vi "FiltroHSV.vi"(8 "error in (no error)":errorcluster, 11 "Refnum in":T1) -> (3 "Array":u32[][](array[numeric]))   [LabVIEW 2021]
uses:
  <vilib>/vision/Image Controls.llb/IMAQ Image.ctl
  <vilib>/vision/NI_Vision_Development_Module.lvlib
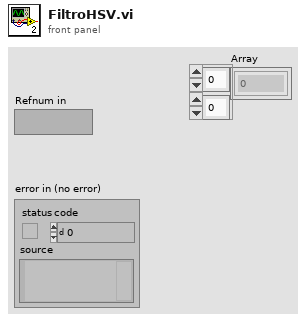
[diagram p1: front panel]
types:
  T1 = typedef "IMAQ Image.ctl" = refnum<image>
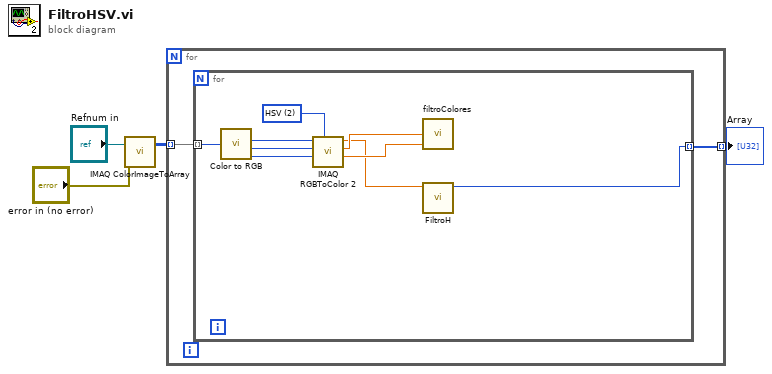
[diagram p0: block diagram]
diagram:
  n1 = call "IMAQ ColorImageToArray"("Image"="Refnum in", "error in (no error)"="error in (no error)") -> ("Image Pixels (U32)"=w1:u32[][])  [unwired: 2 in, 2 out]
  n2 = for {
    tunnel: w1 -> [w6] mode=indexing
    tunnel: [w5] -> w4 mode=indexing
    n3 = for {
      tunnel: w6 -> [w11] mode=indexing
      tunnel: [w7] -> w5 mode=indexing
      w12 = u16 2 items=["RGB", "HSL", "HSV", "HSI", "CIE L*a*b*", "CIE XYZ"] ("Color Mode")
      n4 = call <vilib>:"Color to RGB.vi"("Color"=w11) -> ("R"=w15:u8, "G"=w14:u8, "B"=w13:u8)  [unwired: 1 out]
      n5 = call "IMAQ RGBToColor 2"("Color Mode"=w12, "Blue value"=w13, "Green value"=w14, "Red value"=w15) -> ("Blue or Luma or Val or Inten or Z or b*value"=w10:dbl, "Green or Sat or Y or a* value"=w9:dbl, "Red or Hue or X or L* value"=w8:dbl)  [unwired: 4 in, 1 out]
      n6 = call "filtroColores.vi"("V"=w10, "S"=w9) -> ()  [unwired: 2 in, 2 out]
      n7 = call "FiltroH.vi"("H"=w8) -> ("Color"=w7:u32)  [unwired: 9 in, 1 out]
    }
  }
  "Array" <- w4
